vi "notifiers.vi"() -> ()   [LabVIEW 2019]
doc: "This VI uses a Notifier with a cluster data type to coordinate two While loops. The first loop monitors a 'stop' control and sends a random number to the second loop, which waits for notifications then adds the data points to a chart. The second loop is stopped by the first loop's data."
panel:
  out "Consumer":i32
  out "Producer":i32
  in  "stop":bool
  out "Waveform Chart":dbl(graph)
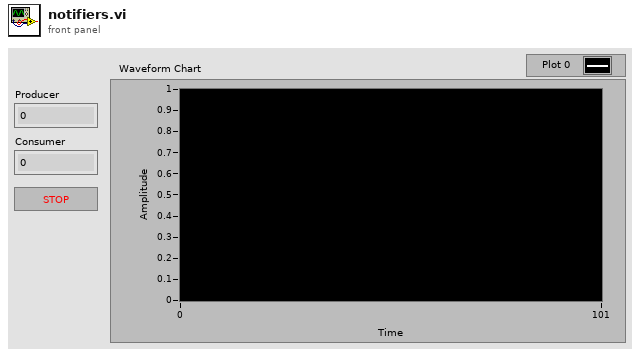
[diagram p1: front panel]
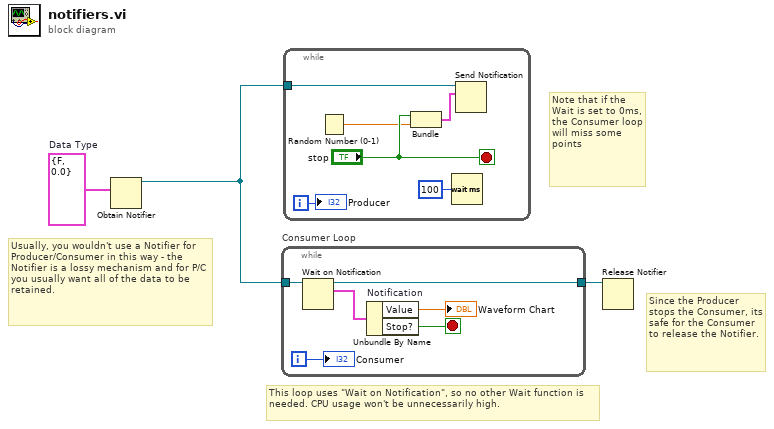
[diagram p0: block diagram]
diagram:
  w3 = cluster{"Stop?":bool, "Value":dbl} {"Stop?"=FALSE, "Value"=0.0}  # Data Type
  # "Since the Producer stops the Consumer, its safe for the Consumer to release the Notifier."
  # "This loop uses \"Wait on Notification\", so no other Wait function is needed. CPU usage won't be unnecessarily high."
  # "Note that if the Wait is set to 0ms, the Consumer loop will miss some points"
  # "Usually, you wouldn't use a Notifier for Producer/Consumer in this way - the Notifier is a lossy mechanism and for P/C you usually want all of the data to be retained."
  n1 = Obtain Notifier(notification data type=w3) -> (notifier out=w2:refnum<notifier>)  [unwired: 3 in, 2 out]
  n2 = while "Consumer Loop" {
    tunnel: w2 -> [w9]
    tunnel: [w4] -> w1
    i -> [w5]
    stop <- w6 stop-if-true
    n3 = Wait on Notification(notifier=w9) -> (notifier out=w4:refnum<notifier>, notification=w8:cluster{"Stop?":bool, "Value":dbl})  [unwired: 3 in, 2 out]
    n4 = Unbundle By Name "Notification"(w8) -> ("Value"=→"Waveform Chart":dbl, "Stop?"=w6:bool)
    "Consumer" <- w5
  }
  n5 = while {
    tunnel: w2 -> [w15]
    i -> [w10]
    stop <- "stop" stop-if-true
    n6 = Random Number (0-1)() -> (number: 0 to 1=w12:dbl)
    n7 = Bundle("stop"="stop", "number: 0 to 1"=w12) -> (w13:cluster{"stop":bool, "number: 0 to 1":dbl})  [unwired: 1 in]
    n8 = Wait (ms)(milliseconds to wait=u32 100) -> ()  [unwired: 1 out]
    n9 = Send Notification(notification=w13, notifier=w15) -> ()  [unwired: 1 in, 2 out]
    "Producer" <- w10
  }
  n10 = Release Notifier(notifier=w1) -> ()  [unwired: 2 in, 3 out]
